vi "Dispach PVMonitors.vi"(8 "Error In":errorcluster, 10 "PV Names (empty)":string[](array[string]), 11 "CS++GUIActor in":refnum<class "CS++GUIActor.lvclass">) -> (0 "Error Out":errorcluster, 3 "CS++GUIActor out":refnum<class "CS++GUIActor.lvclass">)   [LabVIEW 2014, in "CS++GUIActor.lvlib" / "CS++GUIActor.lvclass"]
doc: "Dispatch nested PVMonitor actors according to PV protocoll prefix."
uses:
  CS++GUIActor.lvclass
  CS++GUIActor Messages/Update-PV Msg/Update-PV Msg.lvclass
  CS++PVMonitor/CS++PVMonitor.lvclass
  CS++PVMonitor Messages/CS++PVUpdate Msg/CS++PVUpdate Msg.lvclass/CS++PVUpdate Msg.ctl
  CS++BaseActor/CS++BaseActor.lvclass/CS++BaseActor.ctl
  <vilib>/ActorFramework/Actor/Actor.lvclass/Actor.ctl
  <vilib>/ActorFramework/Message Enqueuer/Message Enqueuer.lvclass/Message Enqueuer.ctl
  Classes/CS++ProcessVariables/ProcessVariable/PV.lvclass/PV.ctl
  Libraries/Base/FGV Action.ctl
  CS++PVMonitor Messages/Register PVs Msg/Register PVs Msg.lvclass/Register PVs Msg.ctl
  CS++GUIActor.lvclass/CS++GUIActor.ctl
  CS++BaseActor/Read Object Name.vi
  CS++BaseActor/Read CS++Factory.vi
  <vilib>/ActorFramework/Message Enqueuer/Init from Existing Queue.vi
  <vilib>/ActorFramework/Message Enqueuer/Enqueue.vi
  Read Associated Actor Name.vi
  <vilib>/ActorFramework/Message Priority Queue/Priority Enqueue.vi
  Classes/CS++ProcessVariables/ProcessVariable/PV.lvclass
  Classes/CS++BaseClasses/Factory/CS++Factory.lvclass
  <vilib>/ActorFramework/Message Enqueuer/Message Enqueuer.lvclass
  CS++PVMonitor Messages/Register PVs Msg/Register PVs Msg.lvclass
  <vilib>/ActorFramework/Actor/Actor.lvclass
  CS++BaseActor/CS++BaseActor.lvclass
  CS++PVMonitor Messages/CS++PVUpdate Msg/CS++PVUpdate Msg.lvclass
  Libraries/Base/CS++Base.lvlib
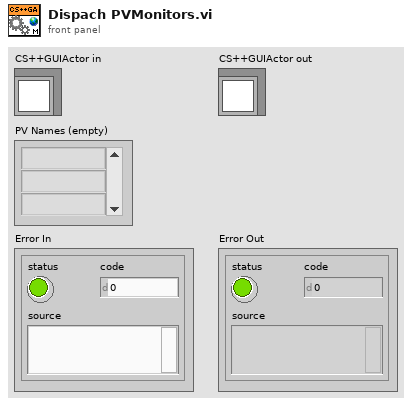
[diagram p1: front panel]
types:
  T1 = cluster{"Msgs":refnum<class "Update-PV Msg.lvclass">[]}[]
  T2 = typedef "CS++Base.lvlib/FGV Action.ctl" = enum16{"add", "replace", "read", "remove", "reset", "get attributes"}
  T3 = cluster{"Msgs":refnum<class "Update-PV Msg.lvclass">[]}
  T4 = cluster{"Self Enqueuer":refnum<class "Message Enqueuer.lvclass">, "Msgs":refnum<class "Update-PV Msg.lvclass">[]}
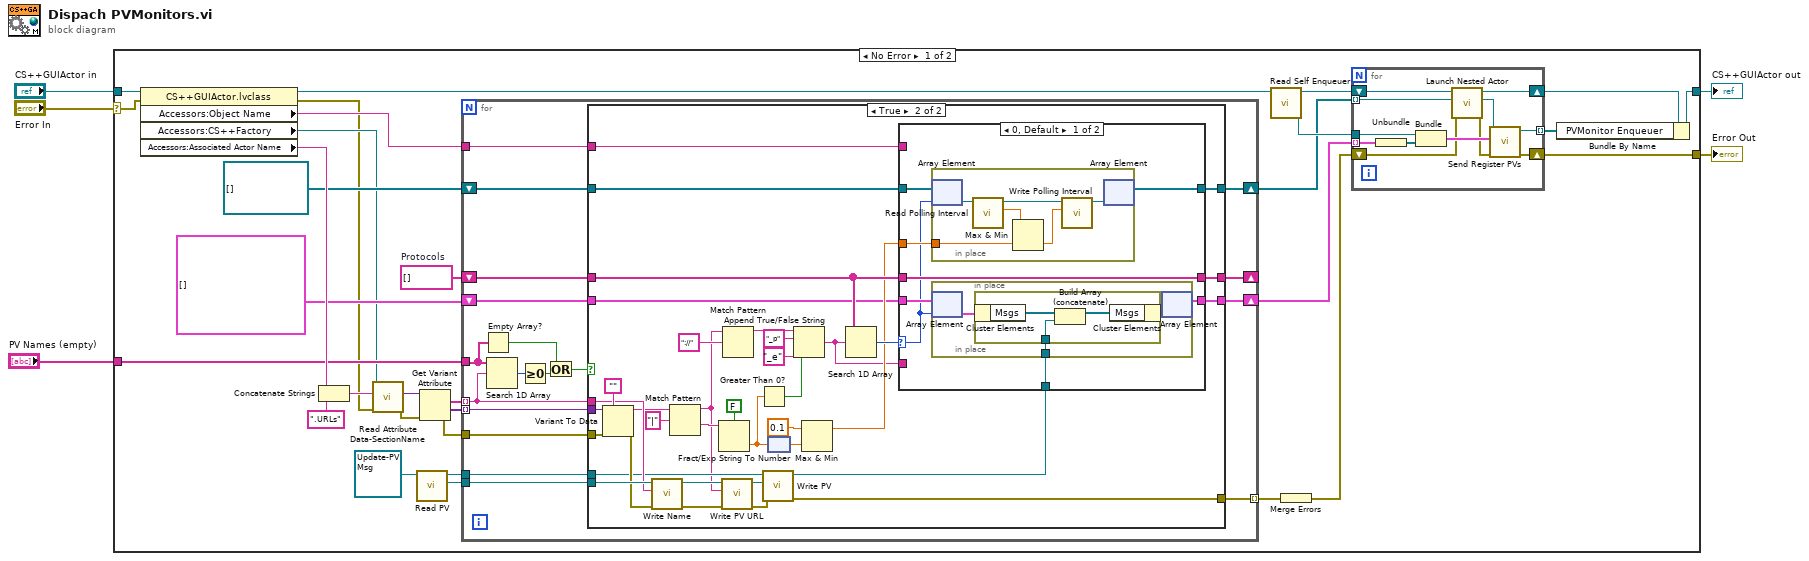
[diagram p0: block diagram]
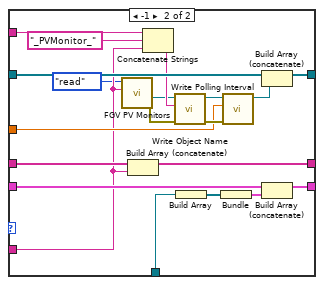
[diagram p3: hidden frame]
diagram:
  n1 = case shown="No Error" "Error In" {
    selector: "Error In" -> [w21 w147]
    tunnel: [w22 w147] -> w4
    tunnel: [w23 w146] -> w2
    tunnel: "CS++GUIActor in" -> [w24 w146]
    tunnel: "PV Names (empty)" -> [w11 _]
    frame No Error {
      w17 = string[] []  # Protocols
      n2 = property class="CS++GUIActor.lvclass"(reference=w24, error in=w21) -> (reference out=w25:refnum<class "CS++GUIActor.lvclass">, error out=w6:errorcluster, "Accessors:Object Name"=w16:string, "Accessors:CS++Factory"=w8:refnum<class "CS++Factory.lvclass">, "Accessors:Associated Actor Name"=w31:string)
      n3 = Concatenate Strings(w31, ".URLs" ("string")) -> (w7:string)
      n4 = call-dynamic "Read Attribute Data-SectionName.vi"("error in (no error)"=w6, "Object Name"=w7, "CS++Factory in"=w8) -> ("error out"=w10:errorcluster, "Attribute Data"=w9:variant)  [unwired: 6 in, 1 out]
      n5 = call "Read PV.vi"("CS++PVUpdate Msg in"=refnum<class "Update-PV Msg.lvclass"> refnum ("CS++DeviceGUIActor.lvlib:Update PV.lvclass")) -> ("PV"=w26:refnum<class "PV.lvclass">, "CS++PVUpdate Msg out"=w27:refnum<class "Update-PV Msg.lvclass">)  [unwired: 8 in, 1 out]
      n6 = Get Variant Attribute(Variant=w9, error in=w10) -> (names=w29:string[], values=w32:variant[], error out=w33:errorcluster)  [unwired: 2 in, 1 out]
      n7 = for {
        tunnel: w32 -> [w65] mode=indexing
        tunnel: w33 -> [w64]
        tunnel: [w61] -> w19 mode=indexing
        tunnel: w27 -> [w62]
        tunnel: w29 -> [w53] mode=indexing
        tunnel: w26 -> [w63]
        shift-right: [w60] -> w15
        shift-left: refnum<class "CS++PVMonitor.lvclass">[] [] -> [w57]
        shift-right: [w59] -> _
        shift-left: w17 -> [w58]
        tunnel: w16 -> [w56]
        shift-right: [w54] -> w12
        shift-left: T1 [] -> [w55]
        tunnel: w11 -> [w52]
        n8 = Empty Array?(array=w52) -> (empty?=w48:bool)
        n9 = Search 1D Array(1D array=w52, element=w53) -> (index of element=w50:i32)  [unwired: 1 in]
        n10 = Greater Or Equal To 0?(x=w50) -> (x >= 0?=w51:bool)
        n11 = Or(x=w48, y=w51) -> (x .or. y?=w49:bool)
        n12 = case shown="True" w49 {
          tunnel: w65 -> [_ w105]
          tunnel: w64 -> [w66 w104]
          tunnel: w63 -> [_ w102]
          tunnel: w53 -> [_ w101]
          tunnel: w62 -> [_ w99]
          tunnel: [w66 w90] -> w61
          tunnel: [w69 w87] -> w60
          tunnel: [w68 w86] -> w59
          tunnel: w58 -> [w68 w84]
          tunnel: w57 -> [w69 w83]
          tunnel: w56 -> [_ w78]
          tunnel: w55 -> [w67 w77]
          tunnel: [w67 w76] -> w54
          frame False {
          }
          frame True {
            n13 = Variant To Data(error in=w104, type="", Variant=w105) -> (data=w98:string, error out=w100:errorcluster)
            n14 = call "Write Name.vi"("error in (no error)"=w100, "Name"=w101, "PV in"=w102) -> ("error out"=w93:errorcluster, "PV out"=w94:refnum<class "PV.lvclass">)  [unwired: 7 in]
            n15 = Match Pattern(string=w98, regular expression="|" ("search string/char (-)")) -> (before substring=w89:string, after substring=w96:string)  [unwired: 1 in, 2 out]
            n16 = Fract/Exp String To Number(use system decimal point (T)=FALSE, string=w96) -> (number=w80:dbl)  [unwired: 2 in, 1 out]
            n17 = call "Write PV URL.vi"("error in (no error)"=w93, "PV URL"=w89, "PV in"=w94) -> ("error out"=w91:errorcluster, "PV out"=w92:refnum<class "PV.lvclass">)  [unwired: 7 in]
            n18 = Match Pattern(string=w89, regular expression="://") -> (before substring=w75:string)  [unwired: 1 in, 3 out]
            n19 = Greater Than 0?(x=w80) -> (x > 0?=w73:bool)
            n20 = call "Write PV.vi"("error in (no error)"=w91, "PV"=w92, "CS++PVUpdate Msg in"=w99) -> ("error out"=w90:errorcluster, "CS++PVUpdate Msg out"=w70:refnum<class "Update-PV Msg.lvclass">)  [unwired: 7 in]
            n21 = node(w80) -> (w82:dbl[unit])
            n22 = Append True/False String(1:w73, 2:"_e" ("false string"), 3:"_p" ("true string"), 4:w75) -> (0:w74:string)
            n23 = Max & Min(x=dbl[unit] 0.1, y=w82) -> (max(x,y)=w79:dbl[unit])  [unwired: 1 out]
            n24 = Search 1D Array(1D array=w84, element=w74) -> (index of element=w85:i32)  [unwired: 1 in]
            n25 = case shown="0, Default" w85 {
              selector: w85 -> [w108 _]
              tunnel: [w111 w145] -> w87
              tunnel: [w113 w144] -> w86
              tunnel: w74 -> [_ w129]
              tunnel: w84 -> [w113 w143]
              tunnel: w83 -> [w112 w142]
              tunnel: w79 -> [w110 w137]
              tunnel: w78 -> [_ w135]
              tunnel: w70 -> [w107 w134]
              tunnel: w77 -> [w109 w132]
              tunnel: [w106 w130] -> w76
              frame 0, Default {
                n26 = in-place {
                  in-place-border: w110 -> [w123]
                  n27 = in-place-array #1(w112, w108) -> (w125:refnum<class "CS++PVMonitor.lvclass">)
                  n28 = call "Read Polling Interval.vi"("CS++BaseActor in"=w125) -> ("Polling Interval"=w124:dbl[unit], "CS++BaseActor out"=w122:refnum<class "CS++PVMonitor.lvclass">)  [unwired: 8 in, 1 out]
                  n29 = Max & Min(x=w124, y=w123) -> (min(x,y)=w121:dbl[unit])  [unwired: 1 out]
                  n30 = call "Write Polling Interval.vi"("Polling Interval"=w121, "CS++BaseActor in"=w122) -> ("CS++BaseActor out"=w120:refnum<class "CS++PVMonitor.lvclass">)  [unwired: 8 in, 1 out]
                  n31 = in-place-array #1(w120) -> (w111:refnum<class "CS++PVMonitor.lvclass">[])  [unwired: 1 out]
                }
                n32 = in-place {
                  in-place-border: w107 -> [w114]
                  n33 = in-place-array #2(w109, w108) -> (w116:T3)
                  n34 = in-place {
                    in-place-border: w114 -> [w118]
                    n35 = in-place-cluster #3(w116) -> ("Msgs"=w119:refnum<class "Update-PV Msg.lvclass">[])
                    n36 = Build Array (concatenate)(w119, w118) -> (w117:refnum<class "Update-PV Msg.lvclass">[])
                    n37 = in-place-cluster #3("Msgs"=w117) -> (w115:T3)
                  }
                  n38 = in-place-array #2(w115) -> (w106:T1)  [unwired: 1 out]
                }
              }
              frame -1 {
                n39 = call "FGV PV Monitors.vi"("PV Monitor"=w129, "Action (read)"=FGV_Action."read") -> ("Error Out"=w126:errorcluster, "CS++PVMonitor"=w128:refnum<class "CS++PVMonitor.lvclass">)  [unwired: 5 in, 3 out]
                n40 = Build Array (concatenate)(w143, w129) -> (w144:string[])
                n41 = Concatenate Strings(w135, "_PVMonitor_" ("Object Name"), w129) -> (w140:string)
                n42 = call "Write Object Name.vi"("error in (no error)"=w126, "Object Name"=w140, "CS++BaseActor in"=w128) -> ("error out"=w138:errorcluster, "CS++BaseActor out"=w139:refnum<class "CS++PVMonitor.lvclass">)  [unwired: 7 in]
                n43 = Build Array(w134) -> (w133:refnum<class "Update-PV Msg.lvclass">[])
                n44 = Bundle(w133) -> (w131:cluster{refnum<class "Update-PV Msg.lvclass">[]})  [unwired: 1 in]
                n45 = call "Write Polling Interval.vi"("error in (no error)"=w138, "Polling Interval"=w137, "CS++BaseActor in"=w139) -> ("CS++BaseActor out"=w136:refnum<class "CS++PVMonitor.lvclass">)  [unwired: 7 in, 1 out]
                n46 = Build Array (concatenate)(w142, w136) -> (w145:refnum<class "CS++PVMonitor.lvclass">[])
                n47 = Build Array (concatenate)(w132, w131) -> (w130:T1)
              }
            }
          }
        }
      }
      n48 = call <vilib>:"Read Self Enqueuer.vi"("Actor"=w25) -> ("Self Enqueuer"=w35:refnum<class "Message Enqueuer.lvclass">)  [unwired: 10 in]
      n49 = Merge Errors(w19) -> (w14:errorcluster)
      n50 = for {
        tunnel: w35 -> [w46]
        tunnel: w15 -> [w37] mode=indexing
        tunnel: w12 -> [w41] mode=indexing
        tunnel: [w38] -> w20 mode=indexing
        shift-right: [w39] -> w22
        shift-left: w14 -> [w43]
        shift-right: [w42] -> w30
        shift-left: w25 -> [w40]
        n51 = Unbundle(w41) -> ("Msgs"=w36:refnum<class "Update-PV Msg.lvclass">[])
        n52 = Bundle("Self Enqueuer"=w46, "Msgs"=w36) -> (w45:T4)  [unwired: 1 in]
        n53 = call <vilib>:"Launch Nested Actor.vi"("error in (no error)"=w43, "Nested Actor"=w37, "Caller Actor in"=w40) -> ("error out"=w44:errorcluster, "Nested Actor's Enqueuer"=w47:refnum<class "Message Enqueuer.lvclass">, "Caller Actor out"=w42:refnum<class "CS++GUIActor.lvclass">)  [unwired: 6 in]
        n54 = call "Send Register PVs.vi"("error in (no error)"=w44, "Register Info"=w45, "Message Enqueuer"=w47) -> ("error out"=w39:errorcluster, "Message Enqueuer out"=w38:refnum<class "Message Enqueuer.lvclass">)  [unwired: 7 in]
      }
      n55 = Bundle By Name(cluster=w30, "PVMonitor Enqueuer"=w20) -> (w23:refnum<class "CS++GUIActor.lvclass">)
    }
    frame Error {
    }
  }
  "Error Out" <- w4
  "CS++GUIActor out" <- w2
